vi "Send Frame.vi"(8 "entrée d'erreur (pas d'erreur)":errorcluster, 9 "Parameter":string, 10 "Cmd":string, 11 "Class Instrument (Default) en entrée":refnum<class "Class Instrument (Default).lvclass">) -> (0 "sortie d'erreur":errorcluster, 3 "Class Instrument (Default) en sortie":refnum<class "Class Instrument (Default).lvclass">)   [LabVIEW 2020, in "Library Test.lvlib" / "P2056_Send_Command_UART.lvclass"]
uses:
  P2056_Send_Command_UART.lvclass
  Instrument/Instrument (Default)/Class Instrument (Default).lvclass
  JSON API/Variant JSON/Variant to JSON.vi
  JSON API/JSON Value/Get Item by name array.vi
  JSON API/JSON Value/JSON Value.lvclass
  P2056_Send_Command_UART.lvclass/P2056_Send_Command_UART.ctl
  JSON API/Get Polymorphic/JSON GetSet.lvlib
  Commun VI/Library Commun.lvlib
  JSON API/Variant JSON/Variant JSON.lvlib
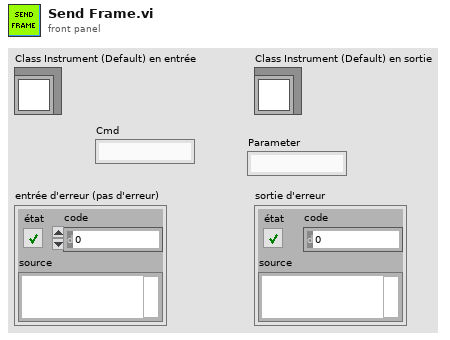
[diagram p1: front panel]
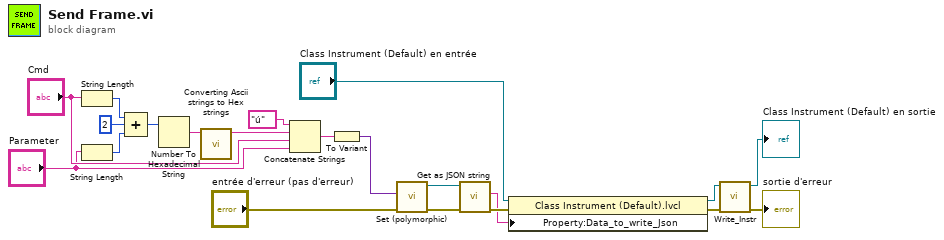
[diagram p0: block diagram]
diagram:
  n1 = String Length(string="Cmd") -> (length=w11:i32)
  n2 = String Length(string="Parameter") -> (length=w1:i32)
  n3 = Compound Arithmetic op=ADD(w11, 2 ("y"), w1) -> (w9:i32)
  n4 = Number To Hexadecimal String(2:w9) -> (0:w4:string)  [unwired: 1 in]
  n5 = call "Converting Ascii strings to Hex strings.vi"("result string"=w4) -> ("Chaîne"=w3:string)  [unwired: 10 in]
  n6 = Concatenate Strings("ú" ("chaîne"), w3, "Cmd", "Parameter") -> (w8:string)
  n7 = To Variant(anything=w8) -> (Variant=w18:variant)
  n8 = call-poly "Set (polymorphic).vi"("error in (no error)"="entrée d'erreur (pas d'erreur)", "Variant"=w18) -> ("error out"=w17:errorcluster, "JSON Value out"=w16:refnum<class "JSON Value.lvclass">)  [unwired: 8 in]
  n9 = call "Get as JSON string.vi"("error in (no error)"=w17, "JSON Value in"=w16) -> ("error out"=w20:errorcluster, "<JSON>"=w19:string)  [unwired: 8 in]
  n10 = property class="Class Instrument (Default).lvcl"(reference="Class Instrument (Default) en entrée", error in=w20, "Property:Data_to_write_Json"=w19) -> (reference out=w15:refnum<class "Class Instrument (Default).lvclass">, error out=w21:errorcluster)
  n11 = call-dynamic "Write_Instr.vi"("error in (no error)"=w21, "Class Multimeter (Default) en entrée"=w15) -> ("error out"=→"sortie d'erreur":errorcluster, "Class Multimeter (Default) en sortie"=→"Class Instrument (Default) en sortie":refnum<class "Class Instrument (Default).lvclass">)  [unwired: 8 in]
